vi "Command Value.vi"(4 "Value":u8 format="%.0b", 5 "Command":T1) -> (7 "Byte":u8 format="%.0b")   [LabVIEW 2020, in "CTI-Peripheral.lvlib" / "HD44780 LCD.lvlib"]
uses:
  HD44780 LCD.lvlib
  Command.ctl
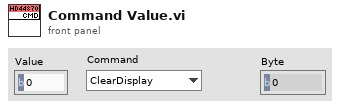
[diagram p1: front panel]
types:
  T1 = typedef "CTI-Peripheral.lvlib/HD44780 LCD.lvlib/Command.ctl" = enum16{"ClearDisplay", "ReturnHome", "EntryModeSet", "DisplayControl", "CursorShift", "FunctionSet", "SetCGRamAddr", "SetDDRamAddr"}
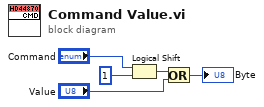
[diagram p0: block diagram]
diagram:
  n1 = Logical Shift(y="Command", x=u8 1 ("Value")) -> (x << y=w4:u8)
  n2 = Or(x=w4, y="Value") -> (x .or. y?=→"Byte":u8)
